vi "Numeric Array To String(I32).vi"(10 "Separator":string, 11 "Numeric Array":i32[](array[numeric])) -> (3 "Result String":string)   [LabVIEW 2016, in "Agilent 3352X Series.lvlib"]
doc: "Phases a I32 numeric array to a serial string separated by specified characters."
uses:
  Agilent 3352X Series.lvlib
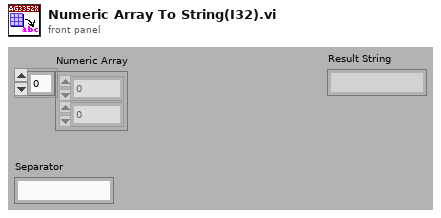
[diagram p1: front panel]
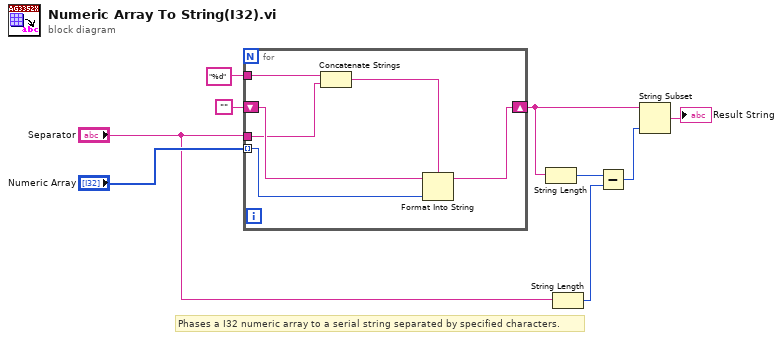
[diagram p0: block diagram]
diagram:
  # "Phases a I32 numeric array to a serial string separated by specified characters."
  n1 = for {
    tunnel: "Numeric Array" -> [w14] mode=indexing
    shift-right: [w15] -> w5
    shift-left: "" ("Empty String Constant") -> [w13]
    tunnel: "Separator" -> [w11]
    tunnel: "%d" ("format string") -> [w10]
    n2 = Concatenate Strings(w10, w11) -> (w12:string)
    n3 = Format Into String(format string=w12, initial string=w13, w14) -> (resulting string=w15:string)  [unwired: 1 in, 1 out]
  }
  n4 = String Length(string=w5) -> (length=w6:i32)
  n5 = String Length(string="Separator") -> (length=w2:i32)
  n6 = Subtract(x=w6, y=w2) -> (x-y=w4:i32)
  n7 = String Subset(string=w5, length (rest)=w4) -> (substring=→"Result String":string)  [unwired: 1 out]
